vi "Set_Amalgamation_Info.vi"(10 "linkerInfo":T2, 11 "Source In":refnum<class "AB_Source.lvclass">) -> (3 "Source Out":refnum<class "AB_Source.lvclass">)   [LabVIEW 2020, in "AB_Source.lvclass"]
uses:
  <vilib>/AppBuilder/AB_Classes/Source/AB_Source.lvclass
  <vilib>/Utility/lvfile.llb/LVFileType.ctl
  <vilib>/AppBuilder/AB_Classes/Source/AB_Source.lvclass/AB_Source.ctl
  <vilib>/Utility/lvfile.llb/NI_FileType.lvlib
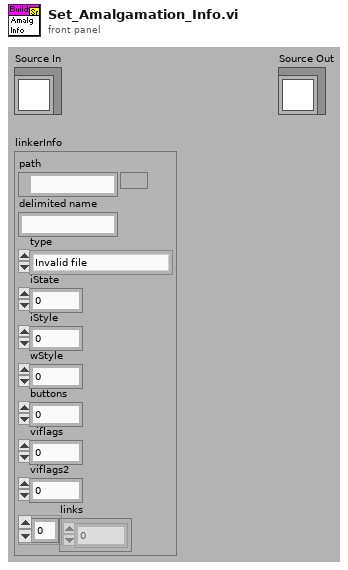
[diagram p1: front panel]
types:
  T1 = typedef "NI_FileType.lvlib/LVFileType.ctl" = enum32{"Invalid file", "Unknown type", "Instrument", "Control", "Polymorphic VI", "Project", "Library", "LVClass", "XControl", "XNode", "Shared library", ".NET assembly", "ActiveX interface", "CIN", "Run-time menu", "Palette menu", "Help file", "LLB", "XNode Edit Dependency", "Class Private Data Control", "Statechart", "MathScript .m file", "Ladder Diagram", "LVLibp", "XNode Build Dependency"}
  T2 = cluster{"path":path, "delimited name":string, "type":T1, "iState":u32, "iStyle":u16, "wStyle":u16, "buttons":u16, "viflags":u32, "viflags2":u32, "links":u32[]}
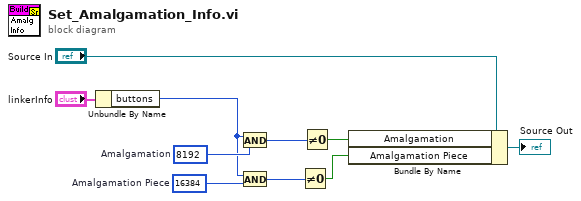
[diagram p0: block diagram]
diagram:
  w9 = u16 16384  # Amalgamation Piece
  w8 = u16 8192  # Amalgamation
  n1 = Unbundle By Name("linkerInfo") -> ("buttons"=w7:u16)
  n2 = And(x=w7, y=w8) -> (x .and. y?=w6:u16)
  n3 = And(x=w7, y=w9) -> (x .and. y?=w5:u16)
  n4 = Not Equal To 0?(x=w5) -> (x != 0?=w3:bool)
  n5 = Not Equal To 0?(x=w6) -> (x != 0?=w2:bool)
  n6 = Bundle By Name(cluster="Source In", "Amalgamation"=w2, "Amalgamation Piece"=w3) -> (→"Source Out":refnum<class "AB_Source.lvclass">)
